vi "STAT2 decode Analog data from PSU.vi"(9 "Temperature base conversion factor":u16=128, 10 "PSU":T1 {"sys register" format="%04x"}) -> (2 "Node Analog value":dbl[](array[numeric]), 3 "Temperature":dbl)   [LabVIEW 2011]
uses:
  LEINmaster/Nodes/PSU stat2.ctl
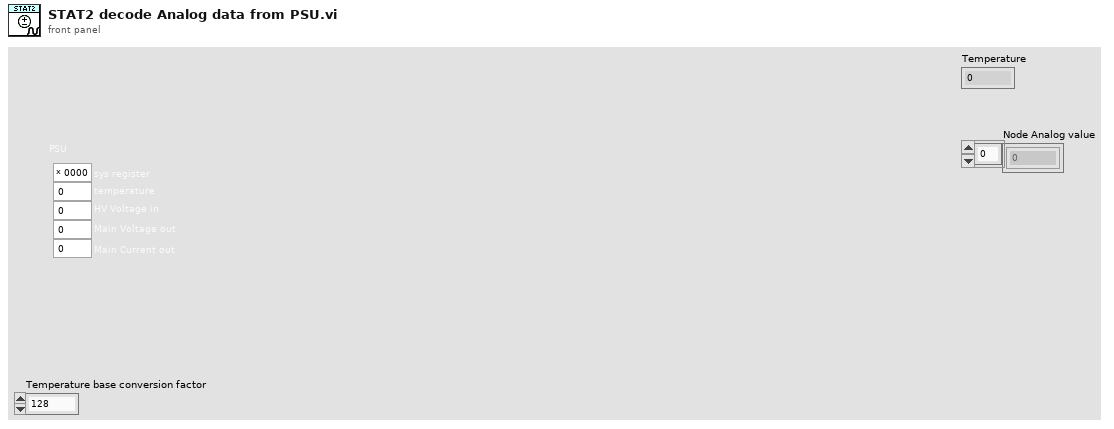
[diagram p1: front panel]
types:
  T1 = typedef "PSU stat2.ctl" = cluster{"sys register":u16, "temperature":u16, "HV Voltage in":u16, "Main Voltage out":u16, "Main Current out":u16}
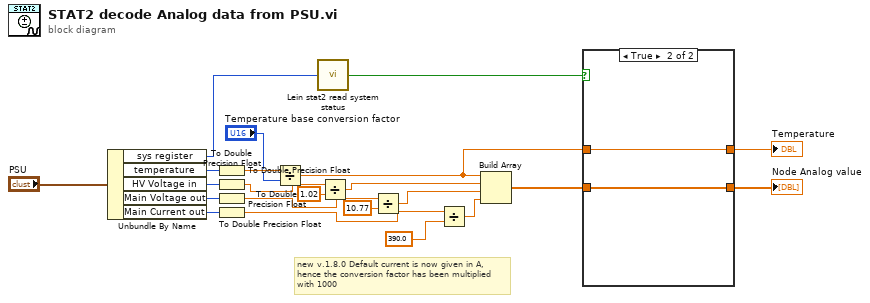
[diagram p0: block diagram]
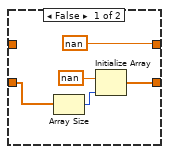
[diagram p2: hidden frame]
diagram:
  # "new v.1.8.0 Default current is now given in A, \nhence the conversion factor has been multiplied\nwith 1000"
  n1 = Unbundle By Name("PSU") -> ("sys register"=w7:u16, "temperature"=w9:u16, "HV Voltage in"=w11:u16, "Main Voltage out"=w12:u16, "Main Current out"=w10:u16)
  n2 = To Double Precision Float(number=w9) -> (double precision float=w13:dbl)
  n3 = To Double Precision Float(number=w11) -> (double precision float=w17:dbl)
  n4 = To Double Precision Float(number=w12) -> (double precision float=w15:dbl)
  n5 = To Double Precision Float(number=w10) -> (double precision float=w22:dbl)
  n6 = Divide(x=w13, y="Temperature base conversion factor") -> (x/y=w3:dbl)
  n7 = call "Lein stat2 read system status.vi"("sys register"=w7) -> ("Connected"=w6:bool)  [unwired: 7 in, 7 out]
  n8 = Divide(x=w17, y=1.02) -> (x/y=w18:dbl)
  n9 = Divide(x=w15, y=10.77) -> (x/y=w16:dbl)
  n10 = Divide(x=w22, y=390.0) -> (x/y=w21:dbl)
  n11 = Build Array(w3, w18, w16, w21) -> (w5:dbl[])
  n12 = case shown="True" w6 {
    tunnel: [w24 w29] -> w4
    tunnel: w5 -> [w27 w29]
    tunnel: [nan ("element") w28] -> w2
    tunnel: w3 -> [_ w28]
    frame False {
      n13 = Array Size(array=w27) -> (size(s)=w26:i32)
      n14 = Initialize Array(nan ("element"), w26) -> (w24:dbl[])
    }
    frame True {
    }
  }
  "Node Analog value" <- w4
  "Temperature" <- w2
